vi "Init RvsT device list.vi"(8 "error in (no error)":errorcluster, 11 "Dynamic FP XControl":refnum<vi>) -> (0 "error out":errorcluster, 2 "find list":string[](array[string]), 3 "Dynamic FP XControl out":refnum<vi>)   [LabVIEW 2015]
uses:
  Dynamic FP XControl.xctl
  <vilib>/Instr/_visa.llb/VISA Find Search Mode.ctl
  Device/Read Name.vi
  Multi-Channel Lockin/Lock-in class/NI-DAQ Lockin.lvclass
  Instruments/Instrument/Instrument.lvclass
panel:
  out "Names":string[](array[string])
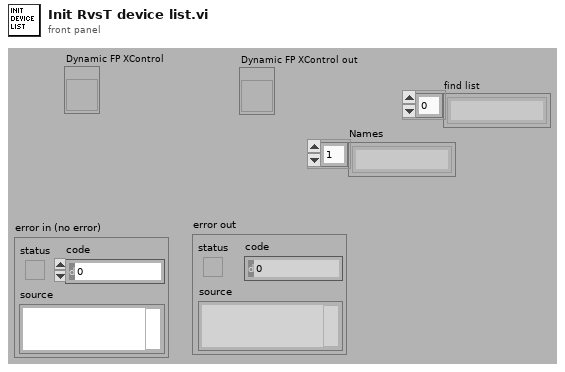
[diagram p1: front panel]
types:
  T1 = typedef "VISA Find Search Mode.ctl" = u32
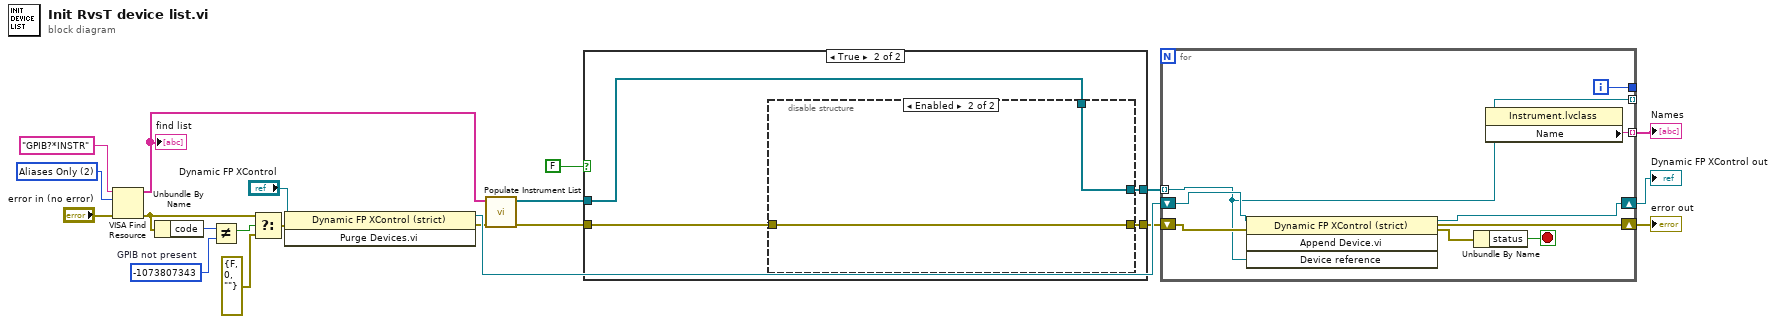
[diagram p0: block diagram]
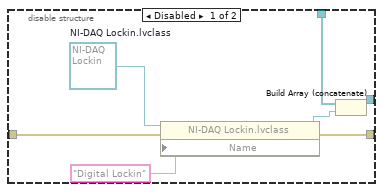
[diagram p3: hidden frame]
diagram:
  w13 = -1073807343  # GPIB not present
  w20 = T1 2 items=["Canonical Names Only"=0, "Aliases Only"=2, "Include Matching Aliases"=3, "Include All Aliases"=4] ("Search Mode")
  n1 = VISA Find Resource(8:"error in (no error)", 10:w20, 11:"GPIB?*INSTR" ("expression (\"?*\")")) -> (0:w11:errorcluster, 3:w19:string[])  [unwired: 1 out]
  "find list" <- w19
  n2 = Unbundle By Name(w11) -> ("code"=w14:i32)
  n3 = Not Equal?(x=w14, y=w13) -> (x != y?=w12:bool)
  n4 = Select(t=w11, s=w12, f=errorcluster {"status"=FALSE, "code"=0, "source"=""}) -> (s? t:f=w8:errorcluster)
  n5 = invoke on="Invoke Node" class="Dynamic FP XControl (strict)" method="Purge Devices.vi"(reference="Dynamic FP XControl", error in=w8) -> (reference out=w17:refnum<vi>, error out=w7:errorcluster)  [unwired: 1 in, 1 out]
  n6 = call "Populate Instrument List.vi"("error in (no error)"=w7, "VISA Resourse Names"=w19) -> ("error out"=w1:errorcluster, "Instrument List"=w4:refnum<class "Instrument.lvclass">[])  [unwired: 2 in, 6 out]
  n7 = case shown="True" FALSE {
    tunnel: w4 -> [w22 w27]
    tunnel: [w22 w26] -> w3
    tunnel: [w23 w25] -> w2
    tunnel: w1 -> [w23 w24]
    frame False {
    }
    frame True {
      n8 = disable-structure shown="Enabled" {
        disable-tunnel: w27 -> [w34 w36]
        disable-tunnel: [w33 w36] -> w26
        disable-tunnel: [w29 w35] -> w25
        disable-tunnel: w24 -> [w28 w35]
        frame Disabled {
          w31 = refnum<class "NI-DAQ Lockin.lvclass"> refnum  # NI-DAQ Lockin.lvclass
          n9 = property class="NI-DAQ Lockin.lvclass"(reference=w31, error in=w28, "Name"="Digital Lockin") -> (reference out=w32:refnum<class "NI-DAQ Lockin.lvclass">, error out=w29:errorcluster)
          n10 = Build Array (concatenate)(w34, w32) -> (w33:refnum<class>[])
        }
        frame Enabled {
        }
      }
    }
  }
  n11 = for {
    tunnel: w3 -> [w37] mode=indexing
    shift-right: [w40] -> w16
    shift-left: w2 -> [w38]
    tunnel: [w37] -> _ mode=indexing
    tunnel: [w43] -> _
    shift-right: [w39] -> w15
    shift-left: w17 -> [w41]
    tunnel: [w42] -> w6 mode=indexing
    i -> [w43]
    stop <- w44 stop-if-true
    n12 = invoke class="Dynamic FP XControl (strict)" method="Append Device.vi"(reference=w41, error in=w38, "Device reference"=w37) -> (reference out=w39:refnum<vi>, error out=w40:errorcluster)  [unwired: 1 in, 2 out]
    n13 = Unbundle By Name(w40) -> ("status"=w44:bool)
    n14 = property class="Instrument.lvclass"(reference=w37) -> ("Name"=w42:string)  [unwired: 1 in, 2 out]
  }
  "error out" <- w16
  "Dynamic FP XControl out" <- w15
  "Names" <- w6
